vi "Calculate Vertex Array.vi"(8 "error in (no error)":errorcluster, 10 "2D Plot Datatype.lvclass in":refnum<class "2D Plot Datatype.lvclass">, 11 "Plot Representation In":T1) -> (0 "error out":errorcluster, 2 "2D Plot Datatype.lvclass out":refnum<class "2D Plot Datatype.lvclass">, 3 "Plot Representation Out":T1)   [LabVIEW 2017, in "2D Plot Datatype.lvclass"]
uses:
  <vilib>/Math Plots/2D Math Plots/2D Plot/2D Plot Datatype/2D Plot Datatype.lvclass
  <vilib>/Math Plots/2D Math Plots/2D Plot/2D Plot/Typedef/Plot Representation.ctl
  <vilib>/Math Plots/2D Math Plots/2D Plot/2D Plot/Typedef/Range Cluster.ctl
  <vilib>/Math Plots/2D Math Plots/2D Plot/2D Plot/2D Plot.lvclass
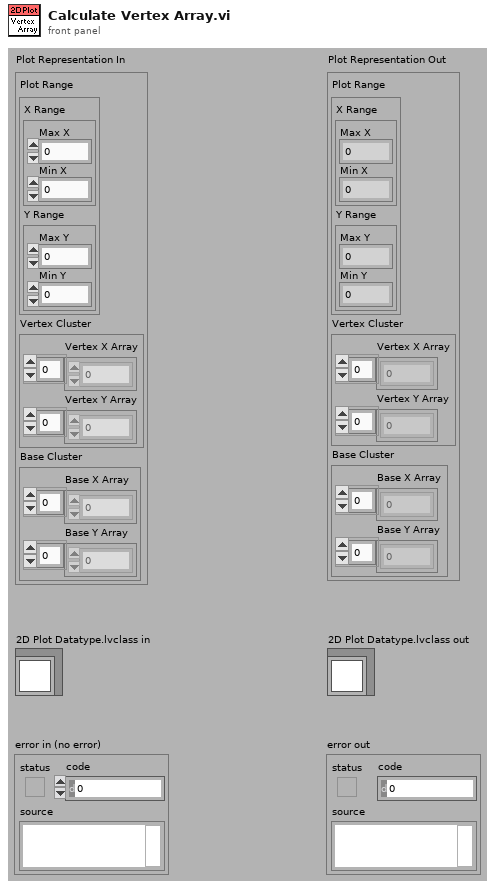
[diagram p1: front panel]
types:
  T1 = typedef "2D Plot.lvclass/Plot Representation.ctl" = cluster{"Plot Range":T2, "Vertex Cluster":cluster{"Vertex X Array":dbl[], "Vertex Y Array":dbl[]}, "Base Cluster":cluster{"Base X Array":dbl[], "Base Y Array":dbl[]}}
  T2 = typedef "2D Plot.lvclass/Range Cluster.ctl" = cluster{"X Range":cluster{"Max X":dbl, "Min X":dbl}, "Y Range":cluster{"Max Y":dbl, "Min Y":dbl}}
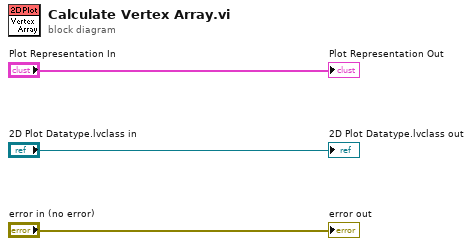
[diagram p0: block diagram]
diagram:
  "2D Plot Datatype.lvclass out" <- "2D Plot Datatype.lvclass in"
  "error out" <- "error in (no error)"
  "Plot Representation Out" <- "Plot Representation In"
